vi "HandleFIFOsetting.vi"(8 "timed out":bool, 11 "Value":u64) -> ()   [LabVIEW 2013]
uses:
  <vilib>/rvi/DataTransferAndStorage/Register/Emulation/niFpgaRegisterEmulationFpgaImpl.vi
  <instcachedir>/0/niFpgaRegisterEmulationFpgaImpl_DCF4BC0110594B98B44A971D60CEEC4D.lvgen/niFpgaRegisterEmulationFpgaImpl_DCF4BC0110594B98B44A971D60CEEC4D_003.vi
  <vilib>/rvi/DataTransferAndStorage/Container/Common/niFpgaContainerGetUniqueNameForEmu.vi
  <instcachedir>/0/niFpgaRegisterEmulationFpgaImpl_DCF4BC0110594B98B44A971D60CEEC4D.lvgen/niFpgaRegisterEmulationFpgaImpl_DCF4BC0110594B98B44A971D60CEEC4D_016.vi
  <instcachedir>/0/niFpgaRegisterEmulationFpgaImpl_DCF4BC0110594B98B44A971D60CEEC4D.lvgen/niFpgaRegisterEmulationFpgaImpl_DCF4BC0110594B98B44A971D60CEEC4D_015.vi
  <instcachedir>/0/niFpgaRegisterEmulationFpgaImpl_DCF4BC0110594B98B44A971D60CEEC4D.lvgen/niFpgaRegisterEmulationFpgaImpl_DCF4BC0110594B98B44A971D60CEEC4D_014.vi
  <instcachedir>/0/niFpgaRegisterEmulationFpgaImpl_DCF4BC0110594B98B44A971D60CEEC4D.lvgen/niFpgaRegisterEmulationFpgaImpl_DCF4BC0110594B98B44A971D60CEEC4D_013.vi
  <instcachedir>/0/niFpgaRegisterEmulationFpgaImpl_DCF4BC0110594B98B44A971D60CEEC4D.lvgen/niFpgaRegisterEmulationFpgaImpl_DCF4BC0110594B98B44A971D60CEEC4D_012.vi
  <instcachedir>/0/niFpgaRegisterEmulationFpgaImpl_DCF4BC0110594B98B44A971D60CEEC4D.lvgen/niFpgaRegisterEmulationFpgaImpl_DCF4BC0110594B98B44A971D60CEEC4D_011.vi
  <instcachedir>/0/niFpgaRegisterEmulationFpgaImpl_DCF4BC0110594B98B44A971D60CEEC4D.lvgen/niFpgaRegisterEmulationFpgaImpl_DCF4BC0110594B98B44A971D60CEEC4D_010.vi
  <instcachedir>/0/niFpgaRegisterEmulationFpgaImpl_DCF4BC0110594B98B44A971D60CEEC4D.lvgen/niFpgaRegisterEmulationFpgaImpl_DCF4BC0110594B98B44A971D60CEEC4D_008.vi
  <instcachedir>/0/niFpgaRegisterEmulationFpgaImpl_DCF4BC0110594B98B44A971D60CEEC4D.lvgen/niFpgaRegisterEmulationFpgaImpl_DCF4BC0110594B98B44A971D60CEEC4D_007.vi
  <instcachedir>/0/niFpgaRegisterEmulationFpgaImpl_DCF4BC0110594B98B44A971D60CEEC4D.lvgen/niFpgaRegisterEmulationFpgaImpl_DCF4BC0110594B98B44A971D60CEEC4D_009.vi
  <instcachedir>/0/niFpgaRegisterEmulationFpgaImpl_DCF4BC0110594B98B44A971D60CEEC4D.lvgen/niFpgaRegisterEmulationFpgaImpl_DCF4BC0110594B98B44A971D60CEEC4D_020.vi
  <instcachedir>/0/niFpgaRegisterEmulationFpgaImpl_DCF4BC0110594B98B44A971D60CEEC4D.lvgen/niFpgaRegisterEmulationFpgaImpl_DCF4BC0110594B98B44A971D60CEEC4D_021.vi
  <vilib>/rvi/DataTransferAndStorage/Container/XNode/niFpgaContainer.xnode
  <vilib>/rvi/DataTransferAndStorage/Register/Emulation/niFpgaRegisterEmulation.vi
  <vilib>/rvi/FXPMathLib/FxpInterpret/XNode/nifxpmath_Interpret.xnode
  fpga_settings.ctl
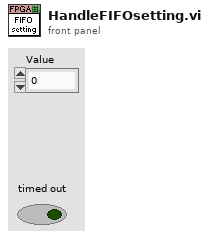
[diagram p1: front panel]
types:
  T1 = typedef "fpga_settings.ctl" = enum16{"Feedback Enable", "New FIR coeffs", "FIR shift", "Enable filter", "Set Downsample", "Downsample", "CIC Gain", "Record length", "Trigger samples", "Quiet time", "a_am", "b_am", "Use fixed delay", "fixed sin_fi", "fixed cos_fi", "Ki*Tau", "Kp", "Kd_Tau", "Fi_start", "Fi_delta", "DC_offs 0", "DC_offs 1", "Ki*Tau am", "Kp am", "Kd_Tau am", "Feedback AM"}
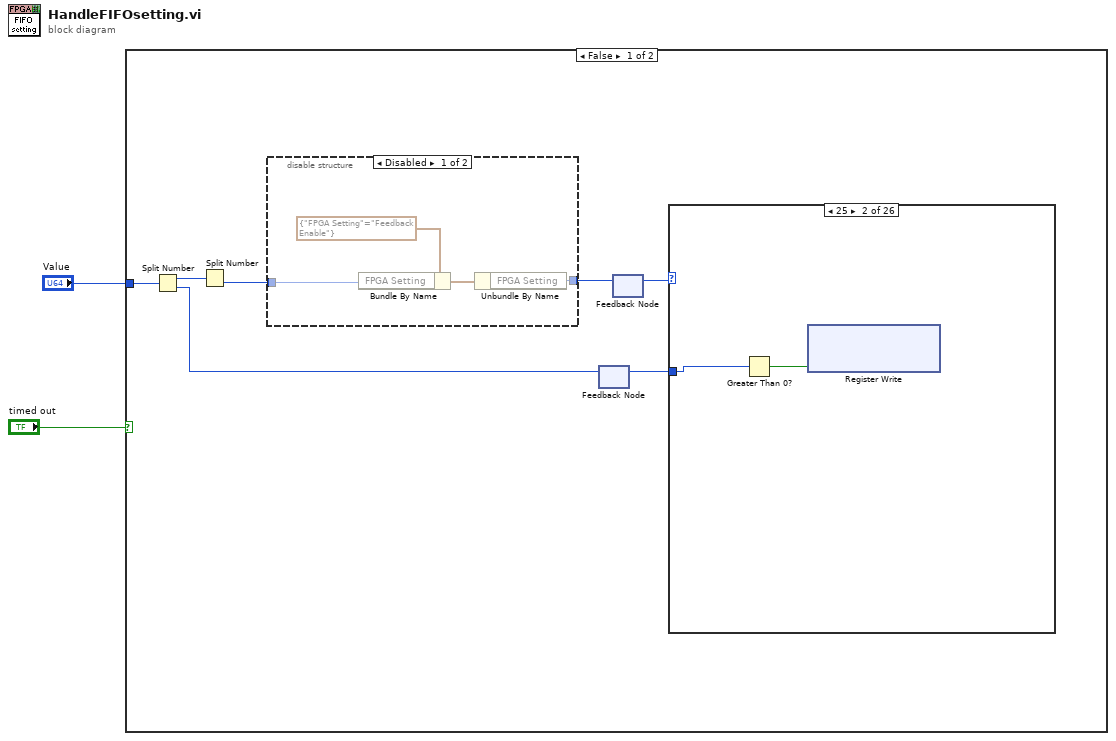
[diagram p0: block diagram]
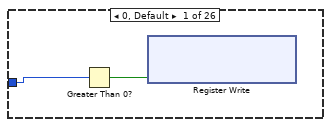
[diagram p3: hidden frame]
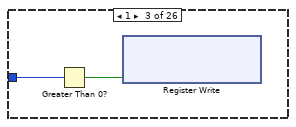
[diagram p4: hidden frame]
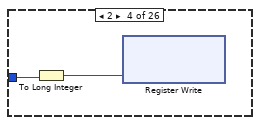
[diagram p5: hidden frame]
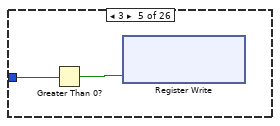
[diagram p6: hidden frame]
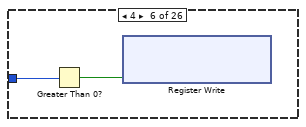
[diagram p7: hidden frame]
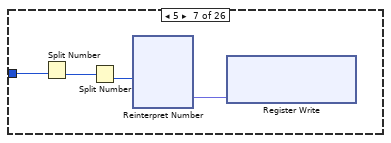
[diagram p8: hidden frame]
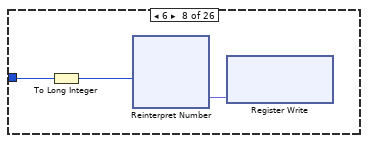
[diagram p9: hidden frame]
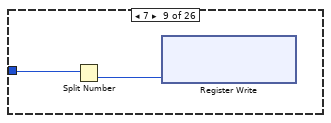
[diagram p10: hidden frame]
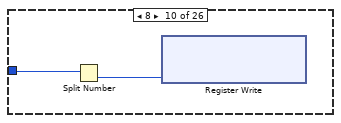
[diagram p11: hidden frame]
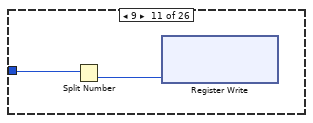
[diagram p12: hidden frame]
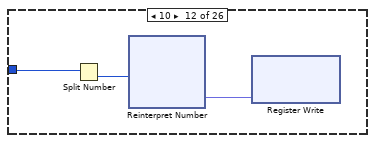
[diagram p13: hidden frame]
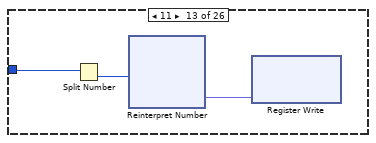
[diagram p14: hidden frame]
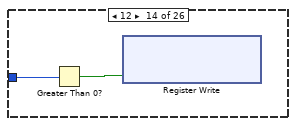
[diagram p15: hidden frame]
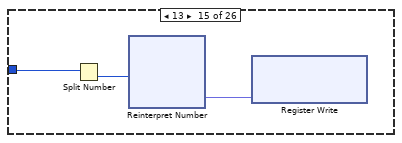
[diagram p16: hidden frame]
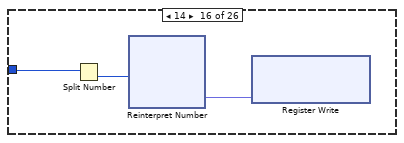
[diagram p17: hidden frame]
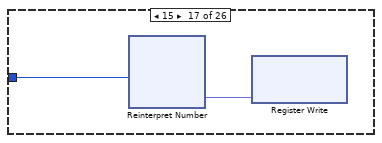
[diagram p18: hidden frame]
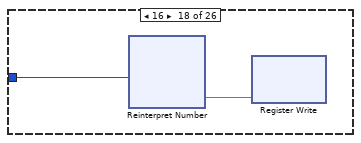
[diagram p19: hidden frame]
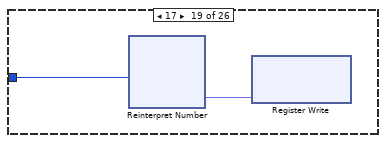
[diagram p20: hidden frame]
diagram:
  n1 = case shown="False" "timed out" {
    tunnel: "Value" -> [w9 _]
    frame False {
      n2 = Split Number(x=w9) -> (hi(x)=w8:u32, lo(x)=w4:u32)
      n3 = Split Number(x=w8) -> (lo(x)=w7:u16)  [unwired: 1 out]
      n4 = disable-structure shown="Disabled" {
        disable-tunnel: [w11 w14] -> w6
        disable-tunnel: w7 -> [w10 w14]
        frame Disabled {
          n5 = Bundle By Name(cluster=cluster{"FPGA Setting":T1} {"FPGA Setting"=enum."Feedback Enable"}, "FPGA Setting"=w10) -> (w12:cluster{"FPGA Setting":T1})
          n6 = Unbundle By Name(w12) -> ("FPGA Setting"=w11:T1)
        }
        frame Enabled {
        }
      }
      n7 = feedback #1() -> (w3:u32)  [unwired: 1 in]
      n8 = feedback-in #1(w4) -> ()
      n9 = feedback #2() -> (w5:u16)  [unwired: 1 in]
      n10 = feedback-in #2(w6) -> ()
      n11 = case shown="25" w5 {
        tunnel: w3 -> [w15 w17 w20 w22 w24 w26 w30 w32 w35 w37 w39 w42 w45 w47 w50 w53 w54 w56 w58 w60 w62 w66 w69 w70 w72 w74]
        frame 0, Default {
          n12 = Greater Than 0?(x=w15) -> (x > 0?=w16:bool)
          n13 = xnode ("Register Write")("Data"=w16) -> ()  [unwired: 1 in, 1 out]
        }
        frame 25 {
          n14 = Greater Than 0?(x=w17) -> (x > 0?=w18:bool)
          n15 = xnode ("Register Write")("Data"=w18) -> ()  [unwired: 1 in, 1 out]
        }
        frame 1 {
          n16 = Greater Than 0?(x=w20) -> (x > 0?=w19:bool)
          n17 = xnode ("Register Write")("Data"=w19) -> ()  [unwired: 1 in, 1 out]
        }
        frame 2 {
          n18 = To Long Integer(number=w22) -> (32bit integer=w21:i32)
          n19 = xnode ("Register Write")("Data"=w21) -> ()  [unwired: 1 in, 1 out]
        }
        frame 3 {
          n20 = Greater Than 0?(x=w24) -> (x > 0?=w23:bool)
          n21 = xnode ("Register Write")("Data"=w23) -> ()  [unwired: 1 in, 1 out]
        }
        frame 4 {
          n22 = Greater Than 0?(x=w26) -> (x > 0?=w25:bool)
          n23 = xnode ("Register Write")("Data"=w25) -> ()  [unwired: 1 in, 1 out]
        }
        frame 5 {
          n24 = Split Number(x=w30) -> (lo(x)=w29:u16)  [unwired: 1 out]
          n25 = Split Number(x=w29) -> (lo(x)=w28:u8)  [unwired: 1 out]
          n26 = xnode "Reinterpret Number"("x"=w28) -> ("y"=w27:fxp<+,8,8>)
          n27 = xnode ("Register Write")("Data"=w27) -> ()  [unwired: 1 in, 1 out]
        }
        frame 6 {
          n28 = To Long Integer(number=w32) -> (32bit integer=w31:i32)
          n29 = xnode "Reinterpret Number"("x"=w31) -> ("y"=w33:fxp<+/-,32,1>)
          n30 = xnode ("Register Write")("Data"=w33) -> ()  [unwired: 1 in, 1 out]
        }
        frame 7 {
          n31 = Split Number(x=w35) -> (lo(x)=w34:u16)  [unwired: 1 out]
          n32 = xnode ("Register Write")("Data"=w34) -> ()  [unwired: 1 in, 1 out]
        }
        frame 8 {
          n33 = Split Number(x=w37) -> (lo(x)=w36:u16)  [unwired: 1 out]
          n34 = xnode ("Register Write")("Data"=w36) -> ()  [unwired: 1 in, 1 out]
        }
        frame 9 {
          n35 = Split Number(x=w39) -> (lo(x)=w38:u16)  [unwired: 1 out]
          n36 = xnode ("Register Write")("Data"=w38) -> ()  [unwired: 1 in, 1 out]
        }
        frame 10 {
          n37 = Split Number(x=w42) -> (lo(x)=w41:u16)  [unwired: 1 out]
          n38 = xnode "Reinterpret Number"("x"=w41) -> ("y"=w40:fxp<+/-,16,2>)
          n39 = xnode ("Register Write")("Data"=w40) -> ()  [unwired: 1 in, 1 out]
        }
        frame 11 {
          n40 = Split Number(x=w45) -> (lo(x)=w44:u16)  [unwired: 1 out]
          n41 = xnode "Reinterpret Number"("x"=w44) -> ("y"=w43:fxp<+/-,16,2>)
          n42 = xnode ("Register Write")("Data"=w43) -> ()  [unwired: 1 in, 1 out]
        }
        frame 12 {
          n43 = Greater Than 0?(x=w47) -> (x > 0?=w46:bool)
          n44 = xnode ("Register Write")("Data"=w46) -> ()  [unwired: 1 in, 1 out]
        }
        frame 13 {
          n45 = Split Number(x=w50) -> (lo(x)=w49:u16)  [unwired: 1 out]
          n46 = xnode "Reinterpret Number"("x"=w49) -> ("y"=w48:fxp<+/-,16,0>)
          n47 = xnode ("Register Write")("Data"=w48) -> ()  [unwired: 1 in, 1 out]
        }
        frame 14 {
          n48 = Split Number(x=w53) -> (lo(x)=w52:u16)  [unwired: 1 out]
          n49 = xnode "Reinterpret Number"("x"=w52) -> ("y"=w51:fxp<+/-,16,0>)
          n50 = xnode ("Register Write")("Data"=w51) -> ()  [unwired: 1 in, 1 out]
        }
        frame 15 {
          n51 = xnode "Reinterpret Number"("x"=w54) -> ("y"=w55:fxp<+/-,32,4>)
          n52 = xnode ("Register Write")("Data"=w55) -> ()  [unwired: 1 in, 1 out]
        }
        frame 16 {
          n53 = xnode "Reinterpret Number"("x"=w56) -> ("y"=w57:fxp<+/-,32,4>)
          n54 = xnode ("Register Write")("Data"=w57) -> ()  [unwired: 1 in, 1 out]
        }
        frame 17 {
          n55 = xnode "Reinterpret Number"("x"=w58) -> ("y"=w59:fxp<+/-,32,4>)
          n56 = xnode ("Register Write")("Data"=w59) -> ()  [unwired: 1 in, 1 out]
        }
        frame 18 {
          n57 = xnode "Reinterpret Number"("x"=w60) -> ("y"=w61:fxp<+/-,32,4>)
          n58 = xnode ("Register Write")("Data"=w61) -> ()  [unwired: 1 in, 1 out]
        }
        frame 19 {
          n59 = xnode "Reinterpret Number"("x"=w62) -> ("y"=w63:fxp<+/-,32,4>)
          n60 = xnode ("Register Write")("Data"=w63) -> ()  [unwired: 1 in, 1 out]
        }
        frame 20 {
          n61 = Split Number(x=w66) -> (lo(x)=w65:u16)  [unwired: 1 out]
          n62 = xnode "Reinterpret Number"("x"=w65) -> ("y"=w64:fxp<+/-,16,14>)
          n63 = xnode ("Register Write")("Data"=w64) -> ()  [unwired: 1 in, 1 out]
        }
        frame 21 {
          n64 = Split Number(x=w69) -> (lo(x)=w68:u16)  [unwired: 1 out]
          n65 = xnode "Reinterpret Number"("x"=w68) -> ("y"=w67:fxp<+/-,16,14>)
          n66 = xnode ("Register Write")("Data"=w67) -> ()  [unwired: 1 in, 1 out]
        }
        frame 22 {
          n67 = xnode "Reinterpret Number"("x"=w70) -> ("y"=w71:fxp<+/-,32,6>)
          n68 = xnode ("Register Write")("Data"=w71) -> ()  [unwired: 1 in, 1 out]
        }
        frame 23 {
          n69 = xnode "Reinterpret Number"("x"=w72) -> ("y"=w73:fxp<+/-,32,6>)
          n70 = xnode ("Register Write")("Data"=w73) -> ()  [unwired: 1 in, 1 out]
        }
        frame 24 {
          n71 = xnode "Reinterpret Number"("x"=w74) -> ("y"=w75:fxp<+/-,32,6>)
          n72 = xnode ("Register Write")("Data"=w75) -> ()  [unwired: 1 in, 1 out]
        }
      }
    }
    frame True {
    }
  }
